vi "Response.vi"(8 "error in (no error)":errorcluster, 11 "Node Ptr":T2 format="%.0x") -> (0 "error out":errorcluster)   [LabVIEW 2020, in "Instrument Addon System Explorer.lvlib"]
uses:
  Instrument Addon System Explorer.lvlib
  <vilib>/NI VeriStand/Custom Device API/Custom Device API.lvlib
  Addon Shared/Instrument Addon Shared.lvlib
  Addon Shared/Types/FG Control.ctl
  <vilib>/NI VeriStand/UI Controls/Single Node Browser/NI_VS UI Single Node Browser.lvlib
  NationalInstruments.VeriStand.SystemStorage
  Addon Shared/SubVIs/Constants.vi
  <vilib>/NI VeriStand/Custom Device API/Custom Device Item Ref.ctl
  Addon Shared/Types/Response Wait Type.ctl
  NationalInstruments.VeriStand.SystemStorageUI
panel:
  in  "Type Value U32":u32=100 caption="Byte Count Value"
  in  "Channel":refnum<k24>(container) caption="Value"
  in  "Use Channel?":bool
  in  "Linkages":i32(listbox)
  in  "MetaData":string(combo) caption="Available Data Channels"
  in  "Response":string caption="Response Format ( Use [] to define a variable )"
  in  "Header 2":cluster{"Section Name":string}={"Section Name"="Response Message Settings"}
  in  "Wait Type":T1
  in  "Type Value DBL":dbl=100.0 caption="Byte Count Value" format="%#_p"
  in  "SHDocVw.IWebBrowser":refnum<k7>(container)
  in  "Header":cluster{"Section Name":string}={"Section Name"="Response Settings"}
  in  "Description":string
  out "Name":string
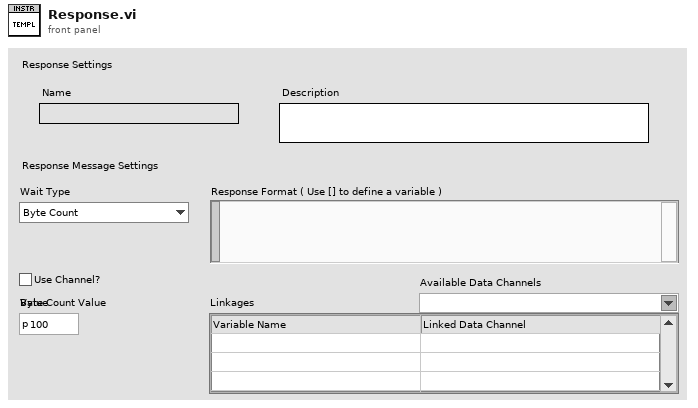
[diagram p1: front panel]
types:
  T1 = typedef "Instrument Addon Shared.lvlib/Response Wait Type.ctl" = enum16{"Byte Count", "Wait sec"}
  T2 = typedef "Custom Device API.lvlib/Custom Device Item Ref.ctl" = u64
  T3 = typedef "Instrument Addon Shared.lvlib/FG Control.ctl" = enum16{"Get", "Set"}
  T4 = typedef "Instrument Addon Shared.lvlib/Response Parameters.ctl" = cluster{"Response":string, "Linked Channels":T5[], "Type Value":dbl, "Wait Type":T1, "Use Channel":bool, "Channel Path":string}
  T5 = typedef "Instrument Addon Shared.lvlib/Linked Channel Cluster.ctl" = cluster{"Variable Name":string, "GUID":string}
  T6 = typedef "Custom Device API.lvlib/Custom Device Item Info.ctl" = cluster{"Name":string, "Is Channel":bool, "GUID":string, "Is Waveform":bool}
  T7 = typedef "Custom Device API.lvlib/Custom Device Commands.ctl" = enum16{"Default", "Item renamed", "Shutdown", "Dynamic button pressed"}
  T8 = typedef "NI_VS UI Single Node Browser.lvlib/Node Ref.ctl" = refnum<k24>
  T9 = typedef "Custom Device API.lvlib/Custom Device Pointer.ctl" = refnum<k24>
  T10 = typedef "LVComboBoxStrsAndValuesArrayTypeDef.ctl" = cluster{"String":string, "Value":string}[]
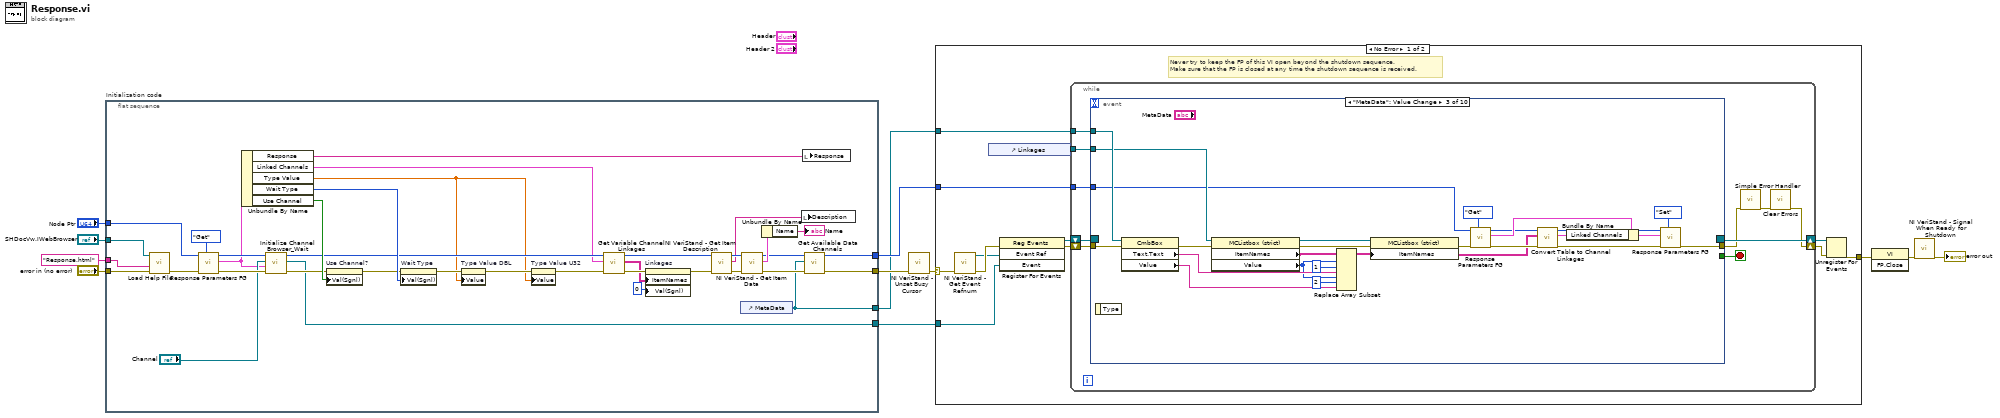
[diagram p0: block diagram]
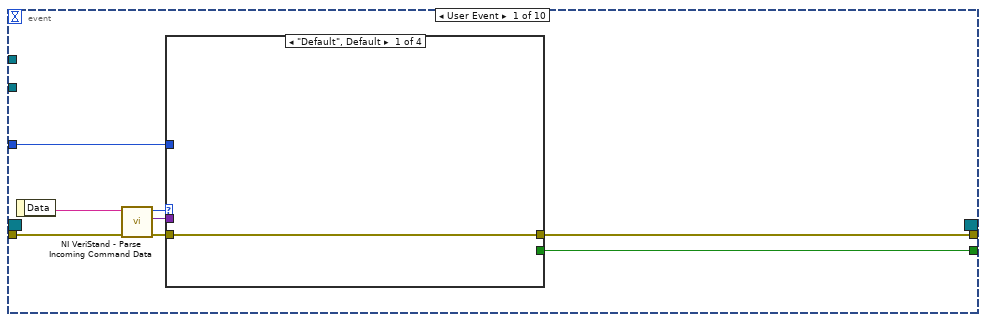
[diagram p2: hidden frame]
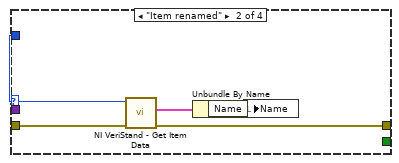
[diagram p3: hidden frame]
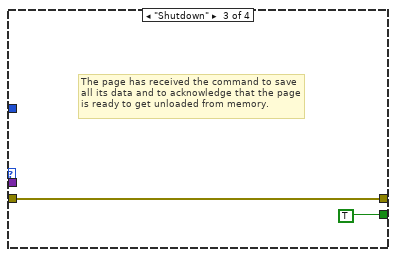
[diagram p4: hidden frame]
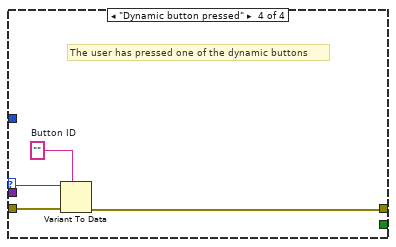
[diagram p5: hidden frame]
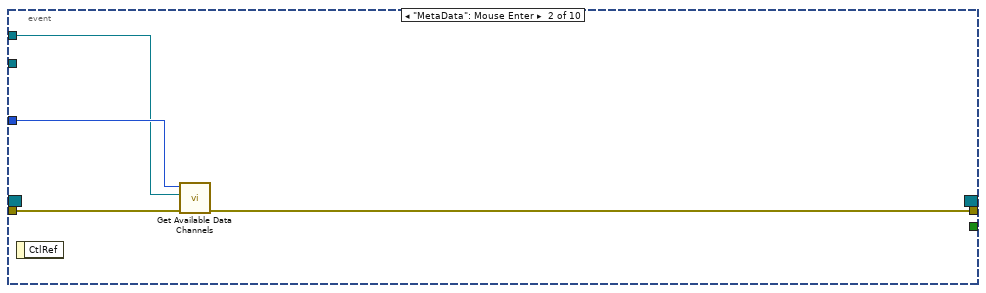
[diagram p6: hidden frame]
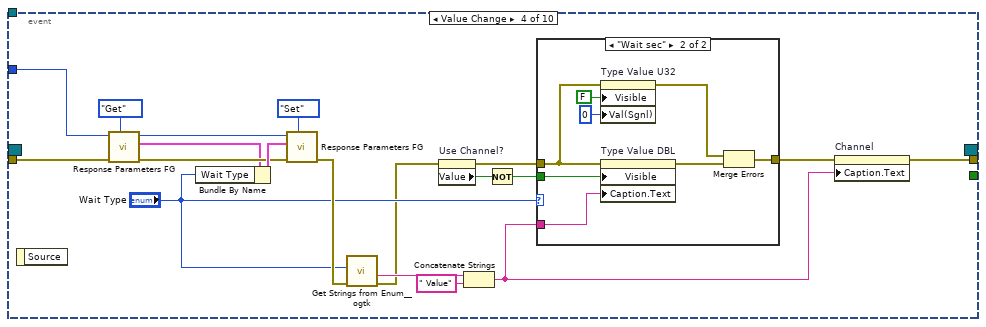
[diagram p7: hidden frame]
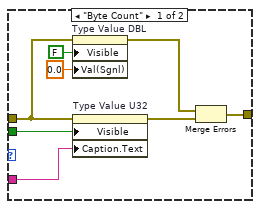
[diagram p8: hidden frame]
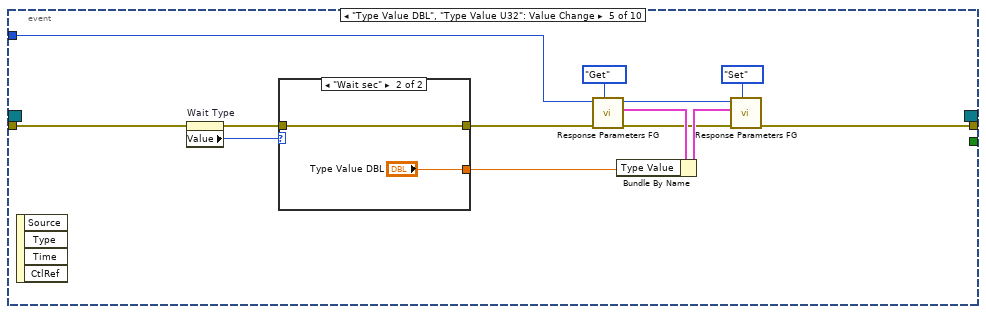
[diagram p9: hidden frame]
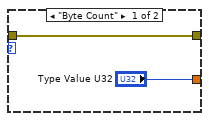
[diagram p10: hidden frame]
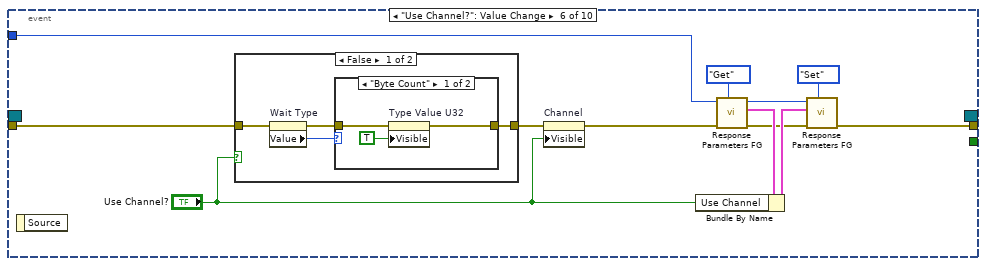
[diagram p11: hidden frame]
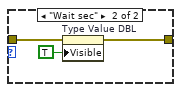
[diagram p12: hidden frame]
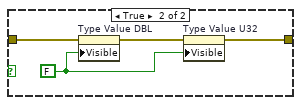
[diagram p13: hidden frame]
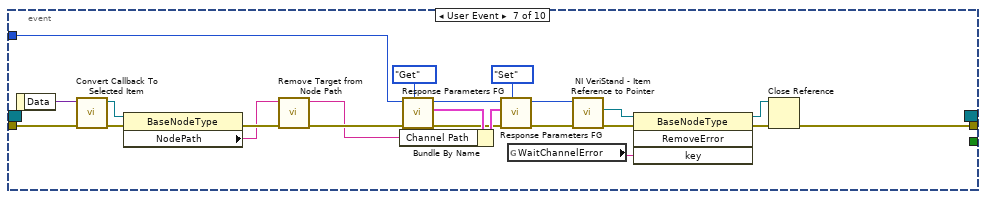
[diagram p14: hidden frame]
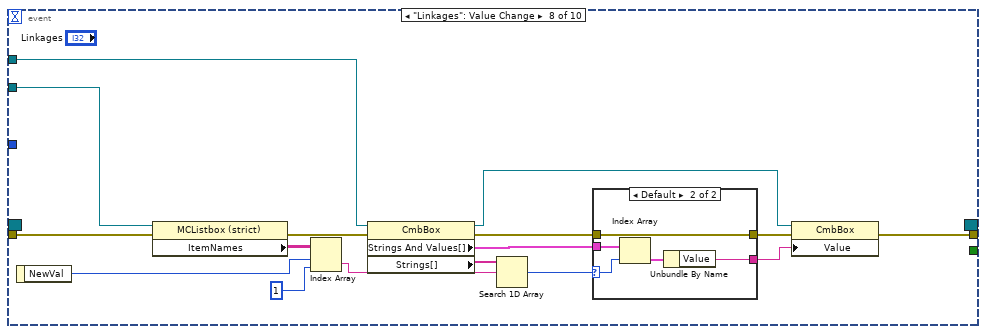
[diagram p15: hidden frame]
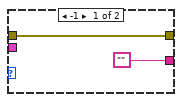
[diagram p16: hidden frame]
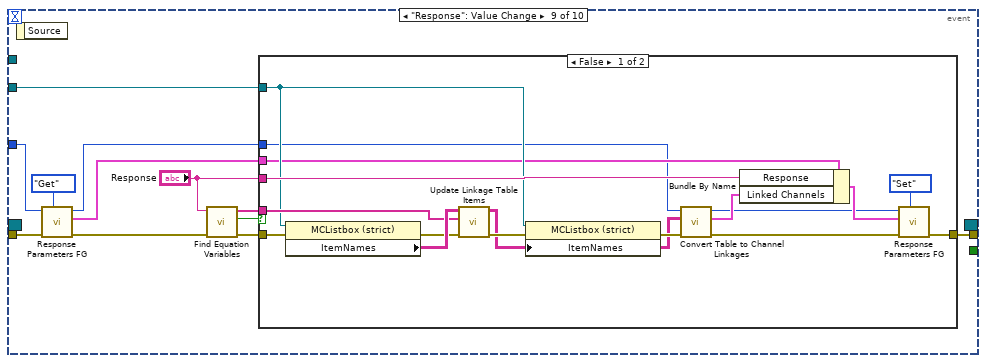
[diagram p17: hidden frame]
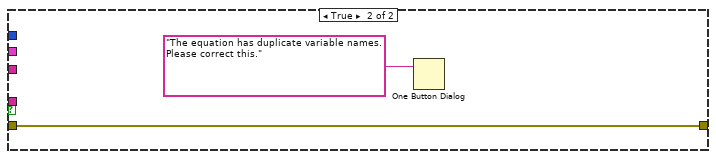
[diagram p18: hidden frame]
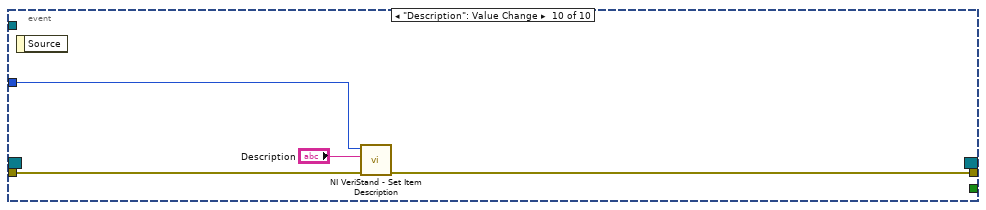
[diagram p19: hidden frame]
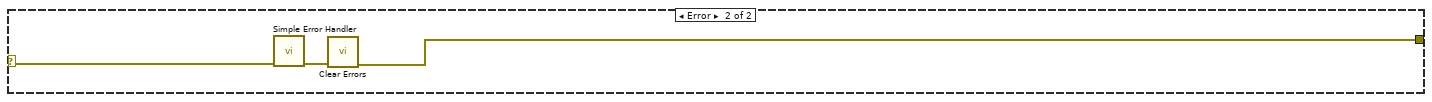
[diagram p20: hidden frame]
diagram:
  n1 = flat-sequence "Initialization code" {
    tunnel: "error in (no error)" -> [w44]
    tunnel: "Node Ptr" -> [w40]
    tunnel: [w34] -> w8
    tunnel: [w32] -> w5
    tunnel: "SHDocVw.IWebBrowser" -> [w43]
    tunnel: "Response.html" ("HTML File") -> [w42]
    tunnel: [w31] -> w2
    tunnel: [w19] -> w1
    frame #0 {
      n2 = call "Load Help File.vi"("error in (no error)"=w44, "HTML File to Load"=w42, "SHDocVw.IWebBrowser2"=w43) -> ("error out"=w41:errorcluster)  [unwired: 8 in]
      n3 = call "Response Parameters FG.vi"("Action"=FG_Control."Get", "error in (no error)"=w41, "Item Ref in"=w40) -> ("error out"=w23:errorcluster, "Response Parameters"=w16:T4, "Item Ref out"=w21:T2)  [unwired: 6 in]
      n4 = Unbundle By Name(w16) -> ("Response"=w36:string, "Linked Channels"=w17:T5[], "Type Value"=w13:dbl, "Wait Type"=w30:T1, "Use Channel"=w24:bool)
      n5 = call "Initialize Channel Browser_Wait.vi"("error in (no error)"=w23, "Reponse Parameters"=w16, ".NET Refnum in"="Channel", "Item Ref in"=w21) -> ("error out"=w22:errorcluster, "Event"=w19:refnum<user-event>, "Item Ref out"=w18:T2)  [unwired: 5 in]
      n6 = property on="Use Channel?" class="Bool (strict)"(error in=w22, "Val(Sgnl)"=w24) -> (error out=w25:errorcluster)  [unwired: 1 in, 1 out]
      n7 = property on="Wait Type" class="Enum (strict)"(error in=w25, "Val(Sgnl)"=w30) -> (error out=w26:errorcluster)  [unwired: 1 in, 1 out]
      n8 = property on="Type Value DBL" class="DigNum (strict)"(error in=w26, "Value"=w13) -> (error out=w15:errorcluster)  [unwired: 1 in, 1 out]
      n9 = property on="Type Value U32" class="DigNum (strict)"(error in=w15, "Value"=w13) -> (error out=w14:errorcluster)  [unwired: 1 in, 1 out]
      n10 = call "Get Variable Channel Linkages.vi"("error in (no error)"=w14, "Linked Channels"=w17, "Item Ref in"=w18) -> ("error out"=w29:errorcluster, "Array"=w27:string[][], "Item Ref out"=w28:T2)  [unwired: 6 in]
      n11 = property on="Linkages" class="MCListbox (strict)"(error in=w29, "ItemNames"=w27, "Val(Sgnl)"=0 ("Value (Signaling)")) -> (error out=w37:errorcluster)  [unwired: 1 in, 1 out]
      n12 = call <vilib>:"NI VeriStand - Get Item Description.vi"("error in (no error)"=w37, "Item Ref in"=w28) -> ("error out"=w47:errorcluster, "Description"=w48:string, "Item Ref out"=w49:T2)  [unwired: 7 out]
      n13 = control-ref of="MetaData"() -> (w31:refnum<vi>)
      n14 = call <vilib>:"NI VeriStand - Get Item Data.vi"("error in (no error)"=w47, "Item Ref in"=w49) -> ("error out"=w35:errorcluster, "Item Info"=w46:T6, "Item Ref out"=w33:T2)  [unwired: 7 out]
      n15 = Unbundle By Name(w46) -> ("Name"=→"Name":string)
      n16 = local write "Description"(w48) -> ()
      n17 = local write "Response"(w36) -> ()
      n18 = call "Get Available Data Channels.vi"("error in (no error)"=w35, "MetaData"=w31, "Item Ref in"=w33) -> ("error out"=w34:errorcluster, "Item Ref out"=w32:T2)  [unwired: 7 in]
    }
  }
  n19 = call <vilib>:"NI VeriStand - Unset Busy Cursor.vi"("error in (no error)"=w8) -> ("error out"=w7:errorcluster)  [unwired: 10 out]
  n20 = case shown="No Error" w7 {
    selector: w7 -> [w53 w282]
    tunnel: [w58 w280] -> w12
    tunnel: w5 -> [w54 _]
    tunnel: w2 -> [w51 _]
    tunnel: w1 -> [w50 _]
    frame No Error {
      # "Never try to keep the FP of this VI open beyond the shutdown sequence.\nMake sure that the FP is closed at any time the shutdown sequence is received."
      n21 = call <vilib>:"NI VeriStand - Get Event Refnum.vi"("error in (no error)"=w53) -> ("error out"=w61:errorcluster, "Event Ref"=w57:refnum<user-event>)  [unwired: 9 out]
      n22 = control-ref of="Linkages"() -> (w52:refnum<vi>)
      n23 = register-events(error in=w61, w57, w50) -> (reference out=w55:refnum<event-registration>, error out=w56:errorcluster)  [unwired: 1 in]
      n24 = while {
        tunnel: w54 -> [w67]
        shift-right: [w64] -> w59
        shift-left: w56 -> [w70]
        shift-right: [w71] -> w60
        shift-left: w55 -> [w69]
        tunnel: w52 -> [w62]
        tunnel: w51 -> [w63]
        stop <- w68 stop-if-true
        n25 = event shown="[2] \"MetaData\": Value Change" {
          selector: w69 -> [_ _ _ _ _ _ _ _ _ _]
          dyn-events: [_ _ _ _ _ _ _ _ _ _] -> w71
          timeout: _ -> [_ _ _ _ _ _ _ _ _ _]
          tunnel: w70 -> [w79 w95 w105 w134 w158 w175 w219 w226 w250 w278]
          tunnel: [w75 _ _ _ _ _ _ _ _ _] -> w68
          tunnel: [w74 w92 w101 w128 w160 w177 w201 w222 w253 w277] -> w66
          tunnel: w67 -> [w73 w94 w102 w135 w163 w176 w211 _ w248 w279]
          tunnel: w63 -> [_ w93 w104 _ _ _ _ w225 _ _]
          tunnel: w62 -> [_ _ w103 _ _ _ _ w224 w252 _]
          event User Event {
            n26 = event-data() -> ("Data"=w78:string)  [unwired: 1 out]
            n27 = call <vilib>:"NI VeriStand - Parse Incoming Command Data.vi"("error in (no error)"=w79, "Incoming data"=w78) -> ("error out"=w77:errorcluster, "Outgoing data"=w72:variant, "Action"=w76:T7)  [unwired: 7 out]
            n28 = case shown="\"Default\", Default" w76 {
              tunnel: w77 -> [w80 w85 w86 w91]
              tunnel: [_ _ TRUE _] -> w75
              tunnel: [w80 w82 w86 w88] -> w74
              tunnel: w73 -> [_ w84 _ _]
              tunnel: w72 -> [_ _ _ w90]
              frame "Default", Default {
              }
              frame "Item renamed" {
                n29 = call <vilib>:"NI VeriStand - Get Item Data.vi"("error in (no error)"=w85, "Item Ref in"=w84) -> ("error out"=w82:errorcluster, "Item Info"=w83:T6)  [unwired: 8 out]
                n30 = Unbundle By Name(w83) -> ("Name"=w81:string)
                n31 = local write "Name"(w81) -> ()
              }
              frame "Shutdown" {
                # "The page has received the command to save all its data and to acknowledge that the page is ready to get unloaded from memory."
              }
              frame "Dynamic button pressed" {
                w89 = ""  # Button ID
                # "The user has pressed one of the dynamic buttons"
                n32 = Variant To Data(error in=w91, type=w89, Variant=w90) -> (error out=w88:errorcluster)  [unwired: 1 out]
              }
            }
          }
          event "MetaData": Mouse Enter {
            n33 = event-data() -> ()  [unwired: 2 out]
            n34 = call "Get Available Data Channels.vi"("error in (no error)"=w95, "MetaData"=w93, "Item Ref in"=w94) -> ("error out"=w92:errorcluster)  [unwired: 7 in, 1 out]
          }
          event "MetaData": Value Change {
            n35 = event-data() -> ()  [unwired: 2 out]
            n36 = property class="CmbBox"(reference=w104, error in=w105) -> (error out=w108:errorcluster, "Text.Text"=w107:string, "Value"=w100:string)  [unwired: 1 out]
            n37 = property class="MCListbox (strict)"(reference=w103, error in=w108) -> (reference out=w118:refnum<vi>, error out=w117:errorcluster, "ItemNames"=w120:string[][], "Value"=w106:i32)
            n38 = Replace Array Subset(array=w120, new element #1=w107, index (row) #1=w106, index (col) #1=1 ("disabled index (col)"), new element #2=w100, index (row) #2=w106, index (col) #2=2 ("disabled index (col)")) -> (w99:string[][])
            n39 = property class="MCListbox (strict)"(reference=w118, error in=w117, "ItemNames"=w99) -> (error out=w112:errorcluster)  [unwired: 1 out]
            n40 = call "Response Parameters FG.vi"("Action"=FG_Control."Get", "error in (no error)"=w112, "Item Ref in"=w102) -> ("error out"=w111:errorcluster, "Response Parameters"=w110:T4, "Item Ref out"=w97:T2)  [unwired: 6 in]
            n41 = call "Convert Table to Channel Linkages.vi"("error in (no error)"=w111, "Item Names"=w99, "Item Ref in"=w97) -> ("error out"=w115:errorcluster, "Linkages"=w98:T5[], "Item Ref out"=w96:T2)  [unwired: 6 in]
            n42 = Bundle By Name(cluster=w110, "Linked Channels"=w98) -> (w114:T4)
            n43 = call "Response Parameters FG.vi"("Action"=FG_Control."Set", "error in (no error)"=w115, "Reponse Parameters"=w114, "Item Ref in"=w96) -> ("error out"=w101:errorcluster)  [unwired: 5 in, 2 out]
          }
          event Value Change {
            n44 = event-data() -> ()  [unwired: 2 out]
            n45 = call "Response Parameters FG.vi"("Action"=FG_Control."Get", "error in (no error)"=w134, "Item Ref in"=w135) -> ("error out"=w133:errorcluster, "Response Parameters"=w126:T4, "Item Ref out"=w136:T2)  [unwired: 6 in]
            n46 = Bundle By Name(cluster=w126, "Wait Type"="Wait Type") -> (w138:T4)
            n47 = call "Response Parameters FG.vi"("Action"=FG_Control."Set", "error in (no error)"=w133, "Reponse Parameters"=w138, "Item Ref in"=w136) -> ("error out"=w131:errorcluster)  [unwired: 5 in, 2 out]
            n48 = call <userlib>:"Get Strings from Enum__ogtk.vi"("error in (no error)"=w131, "Enum"="Wait Type") -> ("error out"=w124:errorcluster, "String Value"=w132:string)  [unwired: 6 in, 2 out]
            n49 = property on="Use Channel?" class="Bool (strict)"(error in=w124) -> (error out=w123:errorcluster, "Value"=w122:bool)  [unwired: 1 in, 1 out]
            n50 = Concatenate Strings(w132, " Value" ("string")) -> (w125:string)
            n51 = Not(x=w122) -> (.not. x?=w121:bool)
            n52 = case shown="\"Wait sec\"" "Wait Type" {
              tunnel: w123 -> [w145 w153]
              tunnel: [w144 w152] -> w129
              tunnel: w125 -> [w147 w155]
              tunnel: w121 -> [w140 w149]
              frame "Byte Count" {
                n53 = property on="Type Value DBL" class="DigNum (strict)"(error in=w145, "Visible"=FALSE, "Val(Sgnl)"=0.0 ("Value (Signaling)")) -> (error out=w143:errorcluster)  [unwired: 1 in, 1 out]
                n54 = property on="Type Value U32" class="DigNum (strict)"(error in=w145, "Visible"=w140, "Caption.Text"=w147) -> (error out=w146:errorcluster)  [unwired: 1 in, 1 out]
                n55 = Merge Errors(w143, w146) -> (w144:errorcluster)
              }
              frame "Wait sec" {
                n56 = property on="Type Value U32" class="DigNum (strict)"(error in=w153, "Visible"=FALSE, "Val(Sgnl)"=u32 0 ("Value (Signaling)")) -> (error out=w151:errorcluster)  [unwired: 1 in, 1 out]
                n57 = property on="Type Value DBL" class="DigNum (strict)"(error in=w153, "Visible"=w149, "Caption.Text"=w155) -> (error out=w154:errorcluster)  [unwired: 1 in, 1 out]
                n58 = Merge Errors(w151, w154) -> (w152:errorcluster)
              }
            }
            n59 = property on="Channel" class="AXCont"(error in=w129, "Caption.Text"=w125) -> (error out=w128:errorcluster)  [unwired: 1 in, 1 out]
          }
          event "Type Value DBL", "Type Value U32": Value Change {
            n60 = event-data() -> ()  [unwired: 5 out]
            n61 = property on="Wait Type" class="Enum (strict)"(error in=w158) -> (error out=w156:errorcluster, "Value"=w159:T1)  [unwired: 1 in, 1 out]
            n62 = case shown="\"Wait sec\"" w159 {
              tunnel: ["Type Value U32" "Type Value DBL"] -> w161
              tunnel: [w169 w171] -> w157
              tunnel: w156 -> [w169 w171]
              frame "Byte Count" {
              }
              frame "Wait sec" {
              }
            }
            n63 = call "Response Parameters FG.vi"("Action"=FG_Control."Get", "error in (no error)"=w157, "Item Ref in"=w163) -> ("error out"=w162:errorcluster, "Response Parameters"=w165:T4, "Item Ref out"=w164:T2)  [unwired: 6 in]
            n64 = Bundle By Name(cluster=w165, "Type Value"=w161) -> (w167:T4)
            n65 = call "Response Parameters FG.vi"("Action"=FG_Control."Set", "error in (no error)"=w162, "Reponse Parameters"=w167, "Item Ref in"=w164) -> ("error out"=w160:errorcluster)  [unwired: 5 in, 2 out]
          }
          event "Use Channel?": Value Change {
            n66 = event-data() -> ()  [unwired: 2 out]
            n67 = case shown="False" "Use Channel?" {
              tunnel: w175 -> [w188 w198]
              tunnel: [w185 w196] -> w174
              frame False {
                n68 = property on="Wait Type" class="Enum (strict)"(error in=w188) -> (error out=w186:errorcluster, "Value"=w187:T1)  [unwired: 1 in, 1 out]
                n69 = case shown="\"Byte Count\"" w187 {
                  tunnel: w186 -> [w191 w194]
                  tunnel: [w190 w193] -> w185
                  frame "Byte Count" {
                    n70 = property on="Type Value U32" class="DigNum (strict)"(error in=w191, "Visible"=TRUE) -> (error out=w190:errorcluster)  [unwired: 1 in, 1 out]
                  }
                  frame "Wait sec" {
                    n71 = property on="Type Value DBL" class="DigNum (strict)"(error in=w194, "Visible"=TRUE) -> (error out=w193:errorcluster)  [unwired: 1 in, 1 out]
                  }
                }
              }
              frame True {
                w195 = FALSE ("Visible")
                n72 = property on="Type Value DBL" class="DigNum (strict)"(error in=w198, "Visible"=w195) -> (error out=w197:errorcluster)  [unwired: 1 in, 1 out]
                n73 = property on="Type Value U32" class="DigNum (strict)"(error in=w197, "Visible"=w195) -> (error out=w196:errorcluster)  [unwired: 1 in, 1 out]
              }
            }
            n74 = property on="Channel" class="AXCont"(error in=w174, "Visible"="Use Channel?") -> (error out=w178:errorcluster)  [unwired: 1 in, 1 out]
            n75 = call "Response Parameters FG.vi"("Action"=FG_Control."Get", "error in (no error)"=w178, "Item Ref in"=w176) -> ("error out"=w179:errorcluster, "Response Parameters"=w181:T4, "Item Ref out"=w180:T2)  [unwired: 6 in]
            n76 = Bundle By Name(cluster=w181, "Use Channel"="Use Channel?") -> (w183:T4)
            n77 = call "Response Parameters FG.vi"("Action"=FG_Control."Set", "error in (no error)"=w179, "Reponse Parameters"=w183, "Item Ref in"=w180) -> ("error out"=w177:errorcluster)  [unwired: 5 in, 2 out]
          }
          event User Event {
            n78 = event-data() -> ("Data"=w218:variant)  [unwired: 1 out]
            n79 = call <vilib>:"Convert Callback To Selected Item.vi"("error in"=w219, "Data"=w218) -> ("error out"=w220:errorcluster, "Selected Item"=w221:T8)  [unwired: 8 in]
            n80 = property class="BaseNodeType"(reference=w221, error in=w220) -> (error out=w210:errorcluster, "NodePath"=w209:string)  [unwired: 1 out]
            n81 = call "Remove Target from Node Path.vi"("error in (no error)"=w210, "NodePath"=w209) -> ("error out"=w208:errorcluster, "PathArrayToString"=w207:string)  [unwired: 8 in]
            n82 = call "Response Parameters FG.vi"("Action"=FG_Control."Get", "error in (no error)"=w208, "Item Ref in"=w211) -> ("error out"=w212:errorcluster, "Response Parameters"=w214:T4, "Item Ref out"=w213:T2)  [unwired: 6 in]
            n83 = Bundle By Name(cluster=w214, "Channel Path"=w207) -> (w216:T4)
            n84 = call "Response Parameters FG.vi"("Action"=FG_Control."Set", "error in (no error)"=w212, "Reponse Parameters"=w216, "Item Ref in"=w213) -> ("error out"=w202:errorcluster, "Item Ref out"=w200:T2)  [unwired: 5 in, 1 out]
            n85 = global read "Constants.vi" "WaitChannelError"() -> (w199:string)
            n86 = call <vilib>:"NI VeriStand - Item Reference to Pointer.vi"("error in (no error)"=w202, "Item Ref in"=w200) -> ("error out"=w204:errorcluster, "Node Pointer"=w203:T9)  [unwired: 6 in, 2 out]
            n87 = invoke class="BaseNodeType" method="RemoveError"(reference=w203, error in=w204, "key"=w199) -> (reference out=w206:T9, error out=w205:errorcluster)  [unwired: 1 in, 2 out]
            n88 = Close Reference(reference=w206, error in (no error)=w205) -> (error out=w201:errorcluster)
          }
          event "Linkages": Value Change {
            n89 = event-data() -> ("NewVal"=w223:i32)  [unwired: 1 out]
            n90 = property class="MCListbox (strict)"(reference=w224, error in=w226) -> (error out=w235:errorcluster, "ItemNames"=w237:string[][])  [unwired: 1 out]
            n91 = Index Array(array=w237, index (row)=w223, index (col)=1 ("disabled index (col)")) -> (element=w234:string)
            n92 = property class="CmbBox"(reference=w225, error in=w235) -> (reference out=w230:refnum<vi>, error out=w228:errorcluster, "Strings And Values[]"=w233:T10, "Strings[]"=w227:string[])
            n93 = Search 1D Array(1D array=w227, element=w234) -> (index of element=w231:i32)  [unwired: 1 in]
            n94 = case shown="Default" w231 {
              selector: w231 -> [_ w242]
              tunnel: w233 -> [_ w244]
              tunnel: ["" w240] -> w232
              tunnel: [w239 w241] -> w229
              tunnel: w228 -> [w239 w241]
              frame -1 {
              }
              frame Default {
                n95 = Index Array(array=w244, index=w242) -> (element=w243:cluster{"String":string, "Value":string})
                n96 = Unbundle By Name(w243) -> ("Value"=w240:string)
              }
            }
            n97 = property class="CmbBox"(reference=w230, error in=w229, "Value"=w232) -> (error out=w222:errorcluster)  [unwired: 1 out]
          }
          event "Response": Value Change {
            n98 = event-data() -> ()  [unwired: 2 out]
            n99 = call "Response Parameters FG.vi"("Action"=FG_Control."Get", "error in (no error)"=w250, "Item Ref in"=w248) -> ("error out"=w249:errorcluster, "Response Parameters"=w246:T4, "Item Ref out"=w247:T2)  [unwired: 6 in]
            n100 = call "Find Equation Variables.vi"("error in (no error)"=w249, "Command"="Response") -> ("error out"=w256:errorcluster, "Duplicate?"=w245:bool, "Variables"=w255:string[])  [unwired: 7 in]
            n101 = case shown="False" w245 {
              tunnel: w256 -> [w267 w275]
              tunnel: w255 -> [w266 _]
              tunnel: "Response" -> [w265 _]
              tunnel: [w264 w275] -> w253
              tunnel: w252 -> [w263 _]
              tunnel: w247 -> [w258 _]
              tunnel: w246 -> [w262 _]
              frame False {
                n102 = property class="MCListbox (strict)"(reference=w263, error in=w267) -> (error out=w268:errorcluster, "ItemNames"=w269:string[][])  [unwired: 1 out]
                n103 = call "Update Linkage Table Items.vi"("error in (no error)"=w268, "Variables"=w266, "Item Names"=w269) -> ("error out"=w270:errorcluster, "Item Names"=w260:string[][])  [unwired: 7 in]
                n104 = property class="MCListbox (strict)"(reference=w263, error in=w270, "ItemNames"=w260) -> (error out=w272:errorcluster)  [unwired: 1 out]
                n105 = call "Convert Table to Channel Linkages.vi"("error in (no error)"=w272, "Item Names"=w260, "Item Ref in"=w258) -> ("error out"=w273:errorcluster, "Linkages"=w259:T5[], "Item Ref out"=w257:T2)  [unwired: 6 in]
                n106 = Bundle By Name(cluster=w262, "Response"=w265, "Linked Channels"=w259) -> (w261:T4)
                n107 = call "Response Parameters FG.vi"("Action"=FG_Control."Set", "error in (no error)"=w273, "Reponse Parameters"=w261, "Item Ref in"=w257) -> ("error out"=w264:errorcluster)  [unwired: 5 in, 2 out]
              }
              frame True {
                n108 = One Button Dialog(message="The equation has duplicate variable names.  Please correct this.") -> ()  [unwired: 1 in, 1 out]
              }
            }
          }
          event "Description": Value Change {
            n109 = event-data() -> ()  [unwired: 2 out]
            n110 = call <vilib>:"NI VeriStand - Set Item Description.vi"("error in (no error)"=w278, "Description"="Description", "Item Ref in"=w279) -> ("error out"=w277:errorcluster)  [unwired: 8 out]
          }
        }
        n111 = call <vilib>:"Simple Error Handler.vi"("error in (no error)"=w66) -> ("error out"=w65:errorcluster)  [unwired: 1 in, 7 out]
        n112 = call <vilib>:"Clear Errors.vi"("error in (no error)"=w65) -> ("error out"=w64:errorcluster)  [unwired: 1 in, 5 out]
      }
      n113 = Unregister For Events(event registration refnum=w60, error in=w59) -> (error out=w58:errorcluster)
    }
    frame Error {
      n114 = call <vilib>:"Simple Error Handler.vi"("error in (no error)"=w282) -> ("error out"=w281:errorcluster)  [unwired: 1 in, 7 out]
      n115 = call <vilib>:"Clear Errors.vi"("error in (no error)"=w281) -> ("error out"=w280:errorcluster)  [unwired: 1 in, 5 out]
    }
  }
  n116 = invoke class="VI" method="FP.Close"(error in=w12) -> (error out=w11:errorcluster)  [unwired: 2 in, 2 out]
  n117 = call <vilib>:"NI VeriStand - Signal When Ready for Shutdown.vi"("error in (no error)"=w11) -> ("error out"=→"error out":errorcluster)  [unwired: 10 out]
